vi "XML writer.vi"   [LabVIEW 2013]
uses:
  <vilib>/Utility/sysdir.llb/System Directory Type.ctl
  <vilib>/xml/Load XML File.vi
  <vilib>/xml/Close Reference(Node).vi
  <vilib>/xml/NI_XML.lvlib
  <resource>/objmgr/DOMUserDefRef.rc
  <vilib>/zip/NI_Unzip.lvlib
types:
  T1 = typedef "System Directory Type.ctl" = i32
  T2 = enum32{"invalid app kind", "Development System", "Run Time System", "Student Edition", "Embedded LabVIEW", "Evaluation", "Custom"}
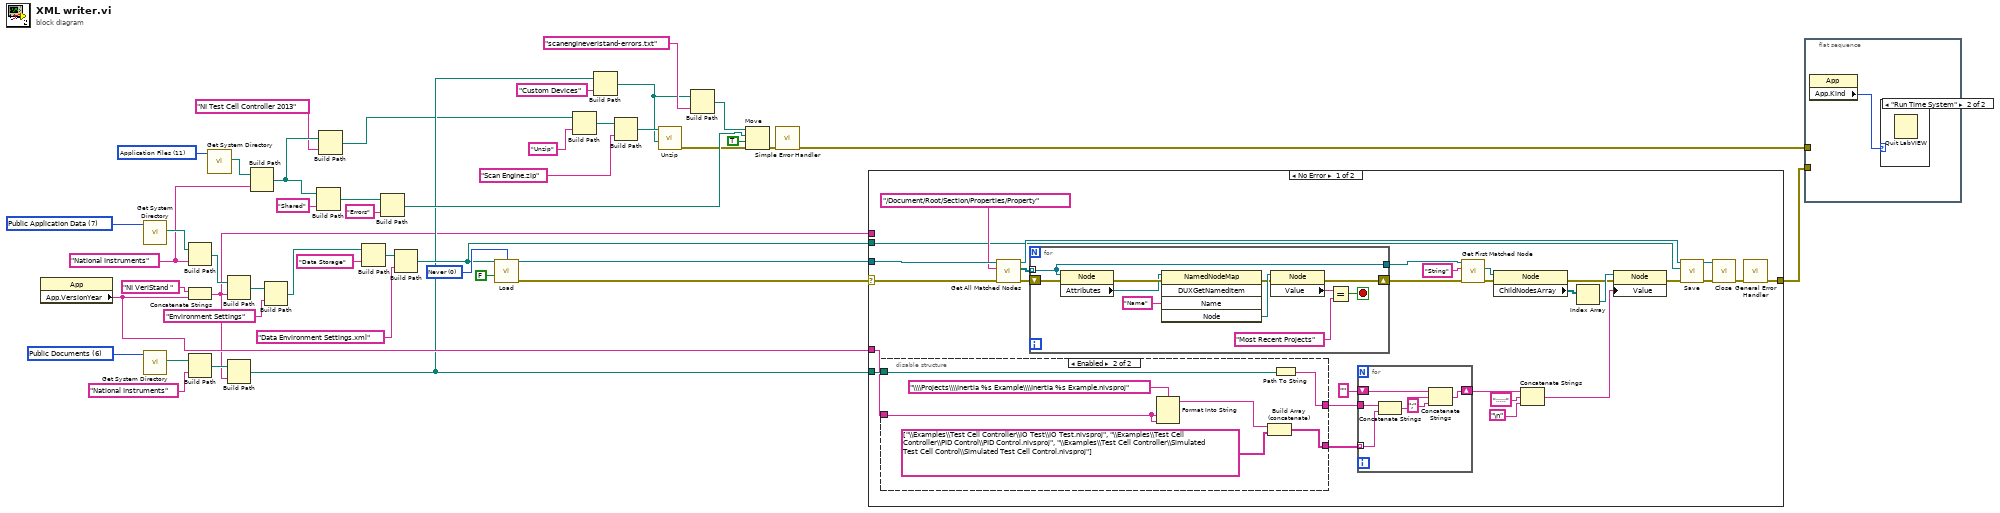
[diagram p0: block diagram]
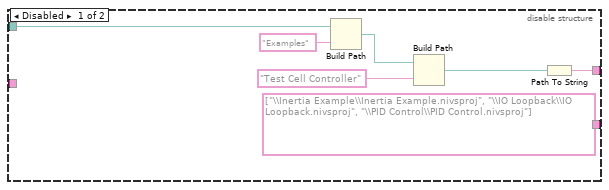
[diagram p3: hidden frame]
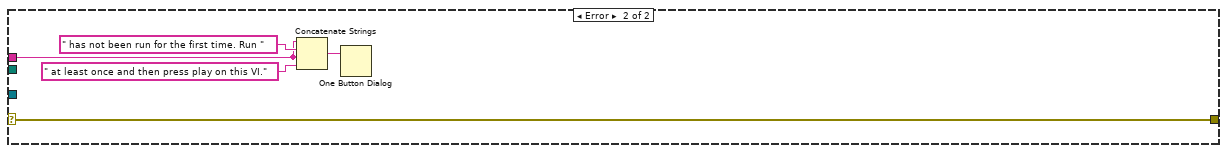
[diagram p4: hidden frame]
diagram:
  w26 = T1 11 items=["User Home", "User Desktop", "User Documents", "User Application Data", "User Preferences", "User Temporary", "Public Documents", "Public Application Data", "Public Preferences", "System Core Libraries", "System Installed Libraries", "Application Files", "Boot Volume Root"] ("system directory type")
  w34 = T1 6 items=["User Home", "User Desktop", "User Documents", "User Application Data", "User Preferences", "User Temporary", "Public Documents", "Public Application Data", "Public Preferences", "System Core Libraries", "System Installed Libraries", "Application Files", "Boot Volume Root"] ("system directory type")
  w37 = 0 items=["Never", "Always", "Auto"] ("validate on load (Auto)")
  w24 = "National Instruments" ("name or relative path")
  w44 = T1 7 items=["User Home", "User Desktop", "User Documents", "User Application Data", "User Preferences", "User Temporary", "Public Documents", "Public Application Data", "Public Preferences", "System Core Libraries", "System Installed Libraries", "Application Files", "Boot Volume Root"] ("system directory type")
  n1 = property class="App"() -> ("App.VersionYear"=w29:string)  [unwired: 2 in, 2 out]
  n2 = call <vilib>:"Get System Directory.vi"("system directory type"=w44) -> ("system directory"=w28:path)  [unwired: 10 in]
  n3 = call <vilib>:"Get System Directory.vi"("system directory type"=w34) -> ("system directory"=w31:path)  [unwired: 10 in]
  n4 = Build Path(base path=w28, name or relative path=w24) -> (appended path=w45:path)
  n5 = Concatenate Strings("NI VeriStand " ("string"), w29) -> (w12:string)
  n6 = Build Path(base path=w31, name or relative path="National Instruments") -> (appended path=w32:path)
  n7 = call <vilib>:"Get System Directory.vi"("system directory type"=w26) -> ("system directory"=w25:path)  [unwired: 10 in]
  n8 = Build Path(base path=w45, name or relative path=w12) -> (appended path=w27:path)
  n9 = Build Path(base path=w32, name or relative path=w12) -> (appended path=w13:path)
  n10 = Build Path(base path=w25, name or relative path=w24) -> (appended path=w10:path)
  n11 = Build Path(base path=w27, name or relative path="Environment Settings") -> (appended path=w41:path)
  n12 = Build Path(base path=w10, name or relative path="Shared") -> (appended path=w22:path)
  n13 = Build Path(base path=w10, name or relative path="NI Test Cell Controller 2013") -> (appended path=w8:path)
  n14 = Build Path(base path=w41, name or relative path="Data Storage") -> (appended path=w39:path)
  n15 = Build Path(base path=w22, name or relative path="Errors") -> (appended path=w14:path)
  n16 = Build Path(base path=w39, name or relative path="Data Environment Settings.xml") -> (appended path=w35:path)
  n17 = call-poly <vilib>:"Load.vi"("path to XML document"=w35, "validate on load (Auto)"=w37, "load external DTD (True)"=FALSE) -> ("DOM document out"=w36:refnum<k20>, "error out"=w7:errorcluster)  [unwired: 10 in, 1 out]
  n18 = Build Path(base path=w8, name or relative path="Unzip") -> (appended path=w17:path)
  n19 = Build Path(base path=w13, name or relative path="Custom Devices") -> (appended path=w11:path)
  n20 = Build Path(base path=w17, name or relative path="Scan Engine.zip") -> (appended path=w19:path)
  n21 = call <vilib>:"Unzip.vi"("Target directory (same as Zip file if empty)"=w11, "Zip file"=w19) -> ("error out"=w4:errorcluster)  [unwired: 7 in, 2 out]
  n22 = Build Path(base path=w11, name or relative path="scanengineveristand-errors.txt") -> (appended path=w5:path)
  n23 = Move(source path=w5, error in=w4, 9:TRUE ("overwrite (F)"), 10:w14) -> (error out=w3:errorcluster)  [unwired: 1 in, 2 out]
  n24 = call <vilib>:"Simple Error Handler.vi"("error in (no error)"=w3) -> ("error out"=w1:errorcluster)  [unwired: 4 in, 4 out]
  n25 = case shown="No Error" w7 {
    selector: w7 -> [w47 w106]
    tunnel: w36 -> [w68 _]
    tunnel: w35 -> [w51 _]
    tunnel: w13 -> [w50 _]
    tunnel: w29 -> [w48 _]
    tunnel: w12 -> [_ w107]
    tunnel: [w46 w106] -> w2
    frame No Error {
      n26 = disable-structure shown="Enabled" {
        disable-tunnel: [string[] ["\\Inertia Example\\Inertia Example.nivsproj", "\\IO Loopback\\IO Loopback.nivsproj", "\\PID Control\\PID Control.nivsproj"] w83] -> w74
        disable-tunnel: [w78 w87] -> w70
        disable-tunnel: w50 -> [w77 w88]
        disable-tunnel: w48 -> [_ w85]
        frame Disabled {
          n27 = Build Path(base path=w77, name or relative path="Examples") -> (appended path=w75:path)
          n28 = Build Path(base path=w75, name or relative path="Test Cell Controller") -> (appended path=w79:path)
          n29 = Path To String(path=w79) -> (string=w78:string)
        }
        frame Enabled {
          n30 = Format Into String(format string="\\\\Projects\\\\Inertia %s Example\\\\Inertia %s Example.nivsproj", w85, w85) -> (resulting string=w82:string)  [unwired: 2 in, 1 out]
          n31 = Build Array (concatenate)(w82, string[] ["\\Examples\\Test Cell Controller\\IO Test\\IO Test.nivsproj", "\\Examples\\Test Cell Controller\\PID Control\\PID Control.nivsproj", "\\Examples\\Test Cell Controller\\Simulated Test Cell Control\\Simulated Test Cell Control.nivsproj"]) -> (w83:string[])
          n32 = Path To String(path=w88) -> (string=w87:string)
        }
      }
      n33 = call <vilib>:"Get All Matched Nodes.vi"("error in (no error)"=w47, "XPath expression"="/Document/Root/Section/Properties/Property", "node in"=w68) -> ("error out"=w66:errorcluster, "node result array"=w65:refnum<k20>[], "node out"=w53:refnum<k20>)  [unwired: 6 in]
      n34 = for {
        shift-right: [w95] -> w62
        shift-left: w66 -> [w92]
        tunnel: w65 -> [w89] mode=indexing
        tunnel: [w89] -> w64
        stop <- w98 stop-if-true
        n35 = property class="Node"(reference=w89, error in=w92) -> (error out=w93:errorcluster, "Attributes"=w90:refnum<k20>)  [unwired: 1 out]
        n36 = invoke class="NamedNodeMap" method="DUXGetNamedItem"(reference=w90, error in=w93, "Name"="Name") -> (error out=w94:errorcluster, "Node"=w96:refnum<k20>)  [unwired: 2 in, 3 out]
        n37 = property class="Node"(reference=w96, error in=w94) -> (error out=w95:errorcluster, "Value"=w91:string)  [unwired: 1 out]
        n38 = Equal?(x=w91, y="Most Recent Projects") -> (x = y?=w98:bool)
      }
      n39 = for {
        tunnel: w74 -> [w104] mode=indexing
        tunnel: w70 -> [w105]
        shift-right: [w100] -> w72
        shift-left: "" -> [w103]
        n40 = Concatenate Strings(w105, w104) -> (w102:string)
        n41 = Concatenate Strings(w103, w102, ";" ("string")) -> (w100:string)
      }
      n42 = call <vilib>:"Get First Matched Node.vi"("error in (no error)"=w62, "XPath expression"="String", "node in"=w64) -> ("error out"=w56:errorcluster, "node result"=w61:refnum<k20>)  [unwired: 6 in, 1 out]
      n43 = property class="Node"(reference=w61, error in=w56) -> (error out=w57:errorcluster, "ChildNodesArray"=w60:refnum<k20>[])  [unwired: 1 out]
      n44 = Concatenate Strings(w72, ";;;;;" ("string"), "\n") -> (w58:string)
      n45 = Index Array(array=w60) -> (element=w59:refnum<k20>)  [unwired: 1 in]
      n46 = property class="Node"(reference=w59, error in=w57, "Value"=w58) -> (error out=w55:errorcluster)  [unwired: 1 out]
      n47 = call <vilib>:"Save.vi"("error in (no error)"=w55, "XML file path"=w51, "DOM document in"=w53) -> ("error out"=w54:errorcluster, "DOM document out"=w52:refnum<k20>)  [unwired: 6 in, 1 out]
      n48 = call-poly <vilib>:"Close.vi"("error in (no error)"=w54, "node"=w52) -> ("error out"=w69:errorcluster)  [unwired: 7 in]
      n49 = call <vilib>:"General Error Handler.vi"("error in (no error)"=w69) -> ("error out"=w46:errorcluster)  [unwired: 10 in, 4 out]
    }
    frame Error {
      n50 = Concatenate Strings(w107, " has not been run for the first time. Run " ("string"), w107, " at least once and then press play on this VI." ("string")) -> (w108:string)
      n51 = One Button Dialog(message=w108) -> ()  [unwired: 1 in, 1 out]
    }
  }
  n52 = flat-sequence {
    tunnel: w2 -> [_]
    tunnel: w1 -> [_]
    frame #0 {
      n53 = property class="App"() -> ("App.Kind"=w111:T2)  [unwired: 2 in, 2 out]
      n54 = case shown="\"Run Time System\"" w111 {
        frame "invalid app kind", Default {
        }
        frame "Run Time System" {
          n55 = Quit LabVIEW() -> ()  [unwired: 1 in]
        }
      }
    }
  }
